vi "Update Clock Wrapper.vi"(8 "error in (no error)":errorcluster, 11 "CIFCorePlugin in":refnum<class "CIFCorePlugin.lvclass">) -> (0 "error out":errorcluster, 3 "CIFCorePlugin out":refnum<class "CIFCorePlugin.lvclass">)   [LabVIEW 2021, in "CIFCorePlugin.lvclass"]
uses:
  CIFCorePlugin.lvclass
  CIFCorePlugin.lvclass/CIFCorePlugin.ctl
  <vilib>/CIF Foundation/CIF Utilities/Time/Typedef/Clock Update.ctl
  <vilib>/CIF Foundation/CIF Utilities/Time/Typedef/Timestamp Pair.ctl
  <vilib>/CIF Foundation/CIF Utilities/Time/Time_CIF_U.lvlib
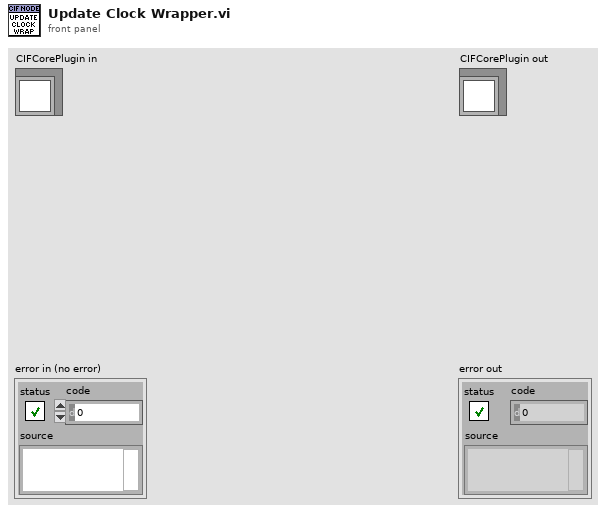
[diagram p1: front panel]
types:
  T1 = typedef "Time_CIF_U.lvlib/Clock Update.ctl" = cluster{"Clock ID":u8, "Timestamp Pair":T2, "reinit":bool, "clock_name":string}
  T2 = typedef "Time_CIF_U.lvlib/Timestamp Pair.ctl" = cluster{"System Time":i64, "External Time":i64}
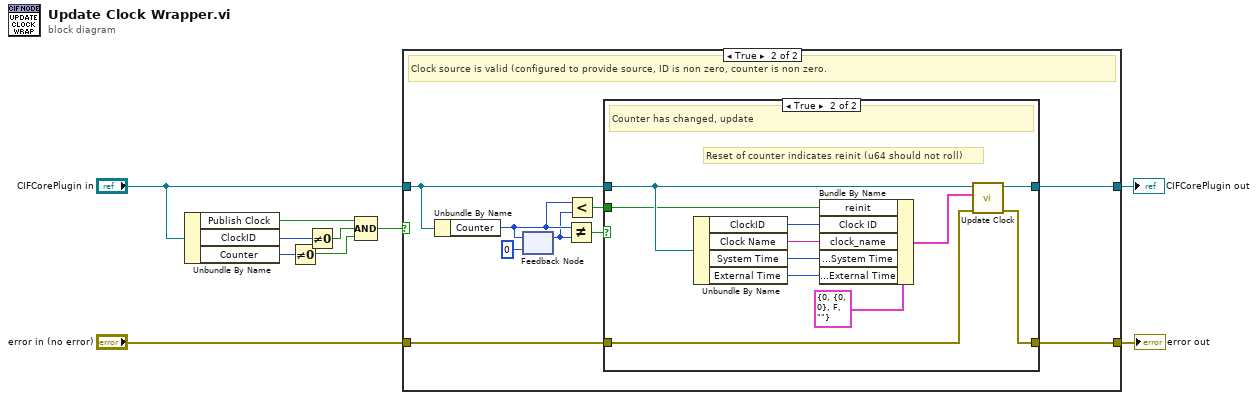
[diagram p0: block diagram]
diagram:
  n1 = Unbundle By Name("CIFCorePlugin in") -> ("Publish Clock"=w6:bool, "ClockID"=w7:u8, "Counter"=w3:u64)
  n2 = Not Equal To 0?(x=w3) -> (x != 0?=w2:bool)
  n3 = Not Equal To 0?(x=w7) -> (x != 0?=w5:bool)
  n4 = Compound Arithmetic op=AND(w6, w5, w2) -> (w4:bool)
  n5 = case shown="True" w4 {
    tunnel: [w11 w21] -> w10
    tunnel: [w12 w20] -> w9
    tunnel: "CIFCorePlugin in" -> [w11 w19]
    tunnel: "error in (no error)" -> [w12 w13]
    frame False {
      # "Not configured as clock source"
    }
    frame True {
      # "Clock source is valid (configured to provide source, ID is non zero, counter is non zero."
      n6 = Unbundle By Name(w19) -> ("Counter"=w16:u64)
      n7 = feedback-in #1(w16) -> ()
      n8 = feedback #1(u64 0 ("Counter")) -> (w15:u64)
      n9 = Not Equal?(x=w16, y=w15) -> (x != y?=w17:bool)
      n10 = Less?(x=w16, y=w15) -> (x < y?=w14:bool)
      n11 = case shown="True" w17 {
        tunnel: [w23 w34] -> w21
        tunnel: [w22 w33] -> w20
        tunnel: w19 -> [w23 w32]
        tunnel: w14 -> [_ w28]
        tunnel: w13 -> [w22 w24]
        frame False {
          # "No clock update"
        }
        frame True {
          # "Reset of counter indicates reinit (u64 should not roll)"
          # "Counter has changed, update"
          n12 = Unbundle By Name(w32) -> ("ClockID"=w30:u8, "Clock Name"=w29:string, "System Time"=w27:i64, "External Time"=w26:i64)
          n13 = Bundle By Name(cluster=T1 {"Clock ID"=0, "Timestamp Pair"={"System Time"=0, "External Time"=0}, "reinit"=FALSE, "clock_name"=""} ("Clock Update"), "reinit"=w28, "Clock ID"=w30, "clock_name"=w29, "Timestamp Pair.System Time"=w27, "Timestamp Pair.External Time"=w26) -> (w25:T1)
          n14 = call "Update Clock.vi"("error in (no error)"=w24, "Clock Update"=w25, "CIFCorePlugin in"=w32) -> ("error out"=w33:errorcluster, "CIFCorePlugin out"=w34:refnum<class "CIFCorePlugin.lvclass">)  [unwired: 7 in]
        }
      }
    }
  }
  "error out" <- w9
  "CIFCorePlugin out" <- w10
